vi "Bitmap Show.vi"(8 "error in (no error)":errorcluster, 10 "Bitmap":refnum<k24>, 11 "PictureBox":refnum<k24>) -> (0 "error out":errorcluster, 2 "Bitmap out":refnum<k24>, 3 "PictureBox out":refnum<k24>)   [LabVIEW 2020, in "SvgDotNet.lvlib"]
uses:
  SvgDotNet.lvlib
  System.Drawing
  System.Windows.Forms
panel:
  # "Connector Pane"
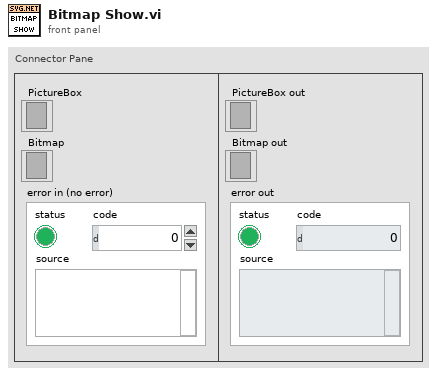
[diagram p1: front panel]
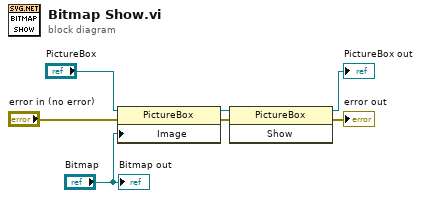
[diagram p0: block diagram]
diagram:
  n1 = property class="PictureBox"(reference="PictureBox", error in="error in (no error)", "Image"="Bitmap") -> (reference out=w3:refnum<k24>, error out=w6:errorcluster)
  n2 = invoke class="PictureBox" method="Show"(reference=w3, error in=w6) -> (reference out=→"PictureBox out":refnum<k24>, error out=→"error out":errorcluster)  [unwired: 1 in, 1 out]
  "Bitmap out" <- "Bitmap"
